vi "Two Ball.vi"   [LabVIEW 2013]
uses:
  <vilib>/Rock Robotics/WPI/Solenoid/WPI_SolenoidValue.ctl
  <vilib>/Rock Robotics/WPI/Solenoid/WPI_SolenoidSetEnum.vi
  Robot Global Data.vi
types:
  T1 = typedef "WPI_SolenoidValue.ctl" = enum16{"Off", "On", "Forward", "Reverse"}
  T2 = typedef "WPI_SolenoidDevRef.ctl" = cluster{"DevStatus":errorcluster, "Solenoid Module":T3, "Forward Solenoid Channel":T4, "Reverse Solenoid Channel":T4}
  T3 = typedef "FPGA_TypedefSolenoidModule.ctl" = enum16{"Solenoid Module 1", "Solenoid Module 2"}
  T4 = typedef "WPI_SolenoidChannel.ctl" = enum8{"Solenoid 1", "Solenoid 2", "Solenoid 3", "Solenoid 4", "Solenoid 5", "Solenoid 6", "Solenoid 7", "Solenoid 8", "Invalid"}
  T5 = typedef "WPI_MotorControlDeviceRef.ctl" = cluster{"DeviceStatus":errorcluster, "Type":enum16{"PWM", "CAN"}, "PWM":cluster{"Digital Module":T6, "PWM Channel":T7, "DeadBand":T8}, "CAN":cluster{"Device Number":u8, "Control Mode":T9, "Semaphore":T10, "Max Vout":dbl}, "Invert":bool, "TransformRef":T11, "InvTransformRef":T11}
  T6 = typedef "FPGA_TypedefDigitalModule.ctl" = enum16{"Digital Module 1", "Digital Module 2"}
  T7 = typedef "FPGA_DIOPWMChannel.ctl" = enum8{"PWM 1", "PWM 2", "PWM 3", "PWM 4", "PWM 5", "PWM 6", "PWM 7", "PWM 8", "PWM 9", "PWM 10", "Invalid"}
  T8 = typedef "WPI_PWMDeadband.ctl" = cluster{"Name":string, "maxPositivePwm":i32, "minPositivePwm":i32, "centerPwm":i32, "maxNegativePwm":i32, "minNegativePwm":i32, "angularRange":u16}
  T9 = typedef "WPI_CANJaguar_ControlMode.ctl" = enum8{"Percent VBus", "Current", "Speed", "Position", "Voltage"}
  T10 = typedef "Semaphore RefNum" = refnum<k1>
  T11 = typedef "WPI_PWMTransform_ConPane.ctl" = refnum<vi>
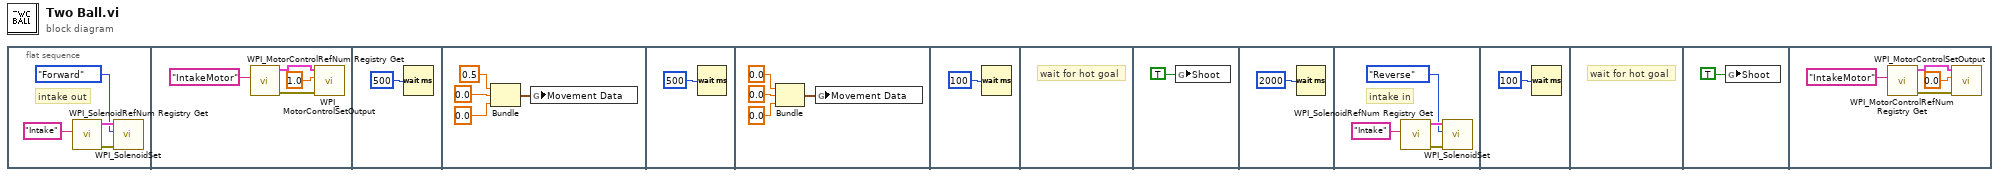
[diagram p0: block diagram]
diagram:
  n1 = flat-sequence {
    frame #0 {
      # "intake out"
      n2 = call <vilib>:"WPI_SolenoidRefNum Registry Get.vi"("refnum name"="Intake") -> ("error out"=w4:errorcluster, "SolenoidDevRef"=w3:T2)  [unwired: 9 in]
      n3 = call-poly <vilib>:"WPI_SolenoidSet.vi"("error in (no error)"=w4, "Value"=WPI_SolenoidValue."Forward", "SolenoidDevRef"=w3) -> ()  [unwired: 7 in, 2 out]
    }
    frame #1 {
      n4 = call <vilib>:"WPI_MotorControlRefNum Registry Get.vi"("refnum name"="IntakeMotor") -> ("error out"=w8:errorcluster, "MotorControlDevRef"=w7:T5)  [unwired: 9 in]
      n5 = call <vilib>:"WPI_MotorControlSetOutput.vi"("error in (no error)"=w8, "Output"=1.0, "MotorControlDevRef"=w7) -> ()  [unwired: 6 in, 3 out]
    }
    frame #2 {
      n6 = Wait (ms)(milliseconds to wait=u32 500) -> ()  [unwired: 1 out]
    }
    frame #3 {
      n7 = Bundle(0.5, 0.0, 0.0) -> (w10:cluster{dbl, dbl, dbl})  [unwired: 1 in]
      n8 = global write "Robot Global Data.vi" "Movement Data"(w10) -> ()
    }
    frame #4 {
      n9 = Wait (ms)(milliseconds to wait=u32 500) -> ()  [unwired: 1 out]
    }
    frame #5 {
      n10 = Bundle(0.0, 0.0, 0.0) -> (w15:cluster{dbl, dbl, dbl})  [unwired: 1 in]
      n11 = global write "Robot Global Data.vi" "Movement Data"(w15) -> ()
    }
    frame #6 {
      n12 = Wait (ms)(milliseconds to wait=u32 100) -> ()  [unwired: 1 out]
    }
    frame #7 {
      # "wait for hot goal"
    }
    frame #8 {
      n13 = global write "Robot Global Data.vi" "Shoot"(TRUE ("Shoot")) -> ()
    }
    frame #9 {
      n14 = Wait (ms)(milliseconds to wait=u32 2000) -> ()  [unwired: 1 out]
    }
    frame #10 {
      # "intake in"
      n15 = call <vilib>:"WPI_SolenoidRefNum Registry Get.vi"("refnum name"="Intake") -> ("error out"=w23:errorcluster, "SolenoidDevRef"=w24:T2)  [unwired: 9 in]
      n16 = call-poly <vilib>:"WPI_SolenoidSet.vi"("error in (no error)"=w23, "Value"=WPI_SolenoidValue."Reverse", "SolenoidDevRef"=w24) -> ()  [unwired: 7 in, 2 out]
    }
    frame #11 {
      n17 = Wait (ms)(milliseconds to wait=u32 100) -> ()  [unwired: 1 out]
    }
    frame #12 {
      # "wait for hot goal"
    }
    frame #13 {
      n18 = global write "Robot Global Data.vi" "Shoot"(TRUE ("Shoot")) -> ()
    }
    frame #14 {
      n19 = call <vilib>:"WPI_MotorControlRefNum Registry Get.vi"("refnum name"="IntakeMotor") -> ("error out"=w31:errorcluster, "MotorControlDevRef"=w28:T5)  [unwired: 9 in]
      n20 = call <vilib>:"WPI_MotorControlSetOutput.vi"("error in (no error)"=w31, "Output"=0.0, "MotorControlDevRef"=w28) -> ()  [unwired: 6 in, 3 out]
    }
  }
